vi "n set duty cycle table.vi"(8 "error in (no error)":errorcluster, 9 "dutycycle":u16, 10 "index":u16, 11 "n":u16) -> (0 "error out":errorcluster)   [LabVIEW 2015, in "SCANalone4x64.lvlib"]
doc: "__declspec(dllimport) void __stdcall n_set_duty_cycle_table(unsigned short n, unsigned short index, unsigned short dutycycle);"
uses:
  <userlib>/SCANalone4x64/SCANalone4x64.lvlib
  <userlib>/SCANalone4x64/SCANalone4x64.dll
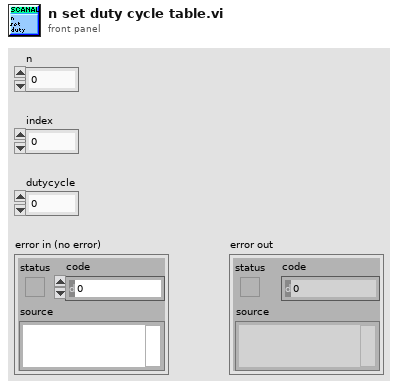
[diagram p1: front panel]
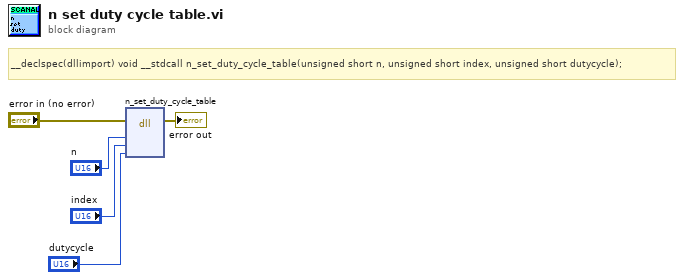
[diagram p0: block diagram]
diagram:
  # "__declspec(dllimport) void __stdcall n_set_duty_cycle_table(unsigned short n, unsigned short index, unsigned short dutycycle);"
  n1 = dll-call lib="C:/Program Files/National Instruments/LabVIEW 2015/user.lib/SCANalone4x64/SCANalone4x64.*" fn="n_set_duty_cycle_table"(error in="error in (no error)", "n"="n", "index"="index", "dutycycle"="dutycycle") -> (error out=→"error out":errorcluster)  [unwired: 6 in, 1 out]
